vi "midi.set.vi"(8 "error in (no error)":errorcluster, 10 "midi.lvclass":refnum<class "midi.lvclass">, 11 "midiPlayer in":refnum<class "midiPlayer.lvclass">) -> (0 "error out":errorcluster, 3 "midiPlayer out":refnum<class "midiPlayer.lvclass">)   [LabVIEW 2020, in "midiPlayer.lvclass"]
uses:
  midiPlayer.lvclass
  midi/midi.lvclass
  midiPlayer.lvclass/midiPlayer.ctl
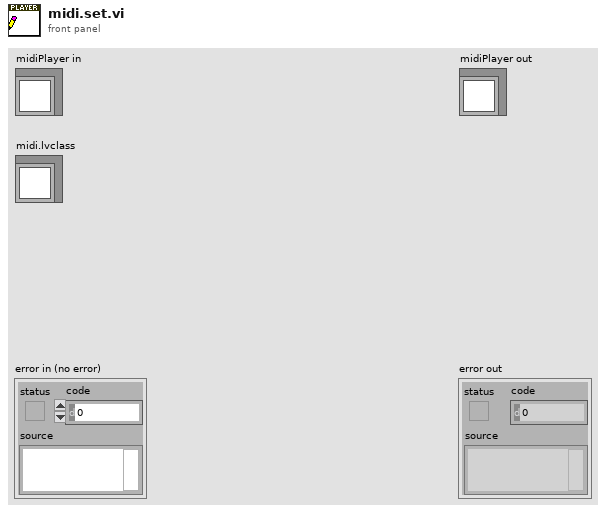
[diagram p1: front panel]
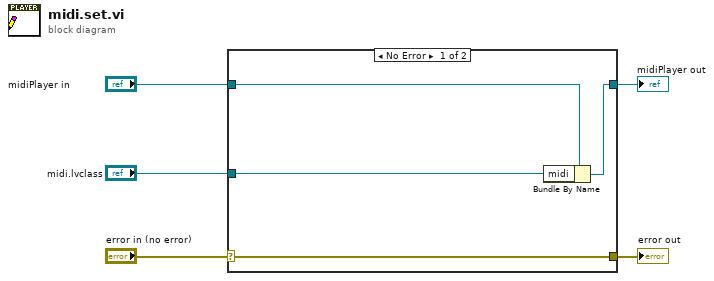
[diagram p0: block diagram]
diagram:
  n1 = case shown="No Error" "error in (no error)" {
    selector: "error in (no error)" -> [w9 w10]
    tunnel: [w9 w10] -> w4
    tunnel: [w7 w11] -> w2
    tunnel: "midiPlayer in" -> [w8 w11]
    tunnel: "midi.lvclass" -> [w6 _]
    frame No Error {
      n2 = Bundle By Name(cluster=w8, "midi"=w6) -> (w7:refnum<class "midiPlayer.lvclass">)
    }
    frame Error {
    }
  }
  "error out" <- w4
  "midiPlayer out" <- w2
